vi "MATLAB Code Calculation Distance.vi"(8 "error in (no error)":errorcluster caption="错误输入（无错误）", 9 "R":dbl, 10 "centre":dbl[](array[numeric]), 11 "Path":path) -> (0 "error out":errorcluster caption="错误输出", 1 "Distance":dbl[](array[numeric]), 2 "Ellipse":dbl[][](array[numeric]), 3 "Circle":dbl[][](array[numeric]))   [LabVIEW 2015, in "Digital Image Processing.lvlib"]
doc: "该模板用于创建子VI。"
uses:
  Digital Image Processing.lvlib
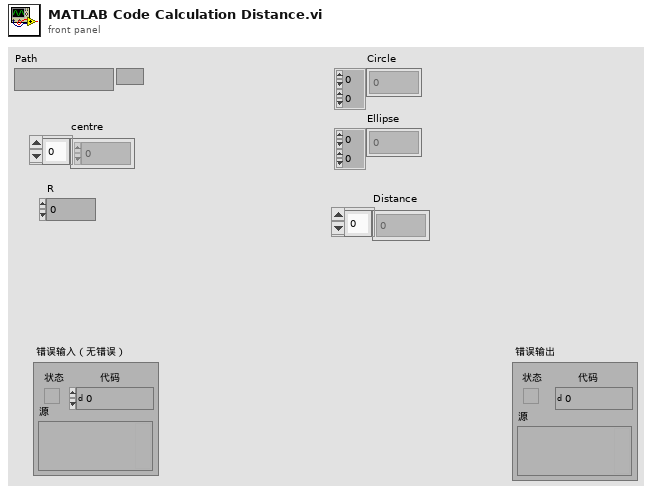
[diagram p1: front panel]
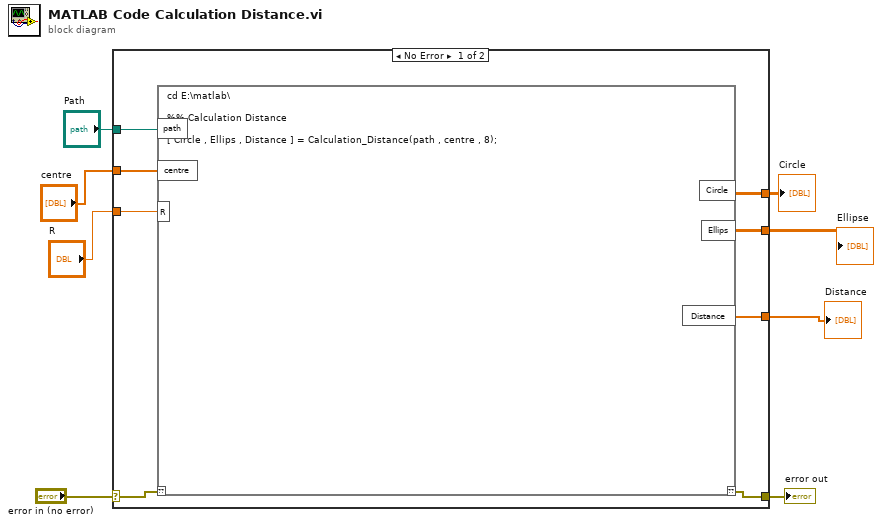
[diagram p0: block diagram]
diagram:
  n1 = case shown="No Error" "error in (no error)" {
    selector: "error in (no error)" -> [w16 w17]
    tunnel: [w15 w17] -> w7
    tunnel: "Path" -> [w14 _]
    tunnel: [w13 _] -> w3
    tunnel: [w12 _] -> w2
    tunnel: [w11 _] -> w1
    tunnel: "centre" -> [w10 _]
    tunnel: "R" -> [w9 _]
    frame No Error {
      n2 = script code="cd E:\\matlab\\\n\n%% Calculation Distance\n\n[ Circle , Ellips , Distance ] = Calculation_Distance(path , centre , 8);"("??"=w16, "path"=w14, "centre"=w10, "R"=w9) -> ("??"=w15:errorcluster, "Circle"=w13:dbl[][], "Ellips"=w12:dbl[][], "Distance"=w11:dbl[])
    }
    frame Error {
    }
  }
  "error out" <- w7
  "Circle" <- w3
  "Ellipse" <- w2
  "Distance" <- w1
